vi "Write Caller Menu Ref.vi"(8 "error in (no error)":errorcluster, 10 "Caller Menu Ref":refnum<k9>, 11 "HIJ Single Cam App Demo in":refnum<class "HIJ IMAQdx Camera Viewer.lvclass">) -> (0 "error out":errorcluster, 3 "HIJ Single Cam App Demo out":refnum<class "HIJ IMAQdx Camera Viewer.lvclass">)   [LabVIEW 2014, in "HIJ IMAQdx Justage Camera w Timer.lvlib" / "HIJ IMAQdx Camera Viewer.lvclass"]
uses:
  HIJ IMAQdx Camera Viewer.lvclass
  HIJ IMAQdx Camera Viewer.lvclass/HIJ IMAQdx Camera Viewer.ctl
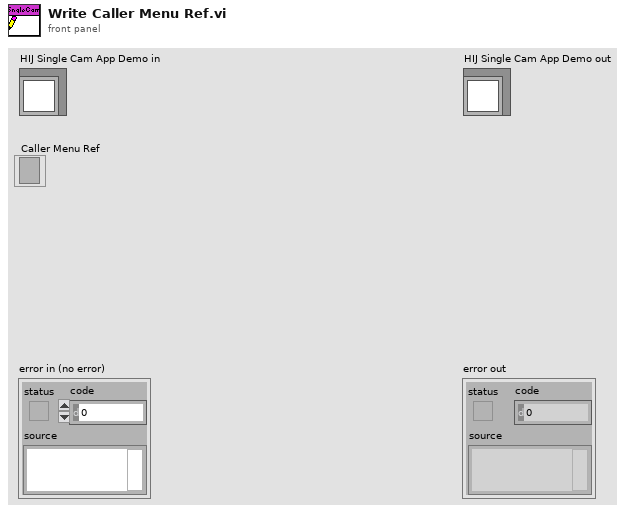
[diagram p1: front panel]
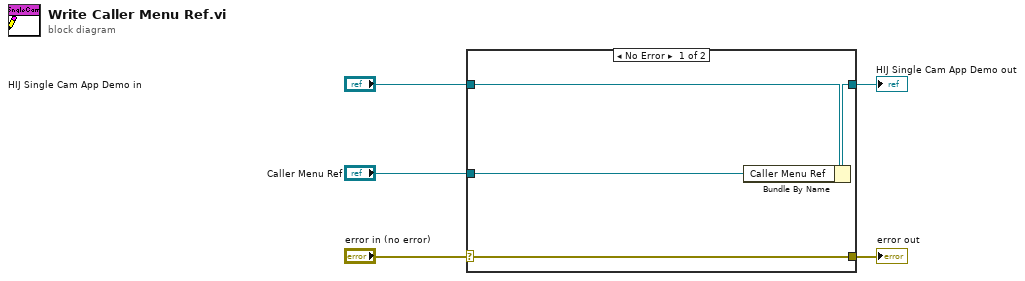
[diagram p0: block diagram]
diagram:
  n1 = case shown="No Error" "error in (no error)" {
    selector: "error in (no error)" -> [w9 w10]
    tunnel: [w9 w10] -> w4
    tunnel: [w7 w11] -> w2
    tunnel: "HIJ Single Cam App Demo in" -> [w8 w11]
    tunnel: "Caller Menu Ref" -> [w6 _]
    frame No Error {
      n2 = Bundle By Name(cluster=w8, "Caller Menu Ref"=w6) -> (w7:refnum<class "HIJ IMAQdx Camera Viewer.lvclass">)
    }
    frame Error {
    }
  }
  "error out" <- w4
  "HIJ Single Cam App Demo out" <- w2
